vi "RTS Run Door Ops.vi"(5 "Delay":bool, 6 "Relay Number":u8=1 min=1 max=3 step=1, 7 "Station 1-8 Data in":T1 {"Station Slide"."Chamber 1-1"."Start Time" format="%<%X\n%x>T"; "Station Slide"."Chamber 1-1"."End Time" format="%<%X\n%x>T"; "Station Slide"."Time Count (s)" format="%.2f"; "Station Cab"."Chamber 1-1"."Start Time" format="%<%X\n%x>T"; "Station Cab"."Chamber 1-1"."End Time" format="%<%X\n%x>T"; "Station Cab"."Time Count (s)" format="%.2f"; "Station Freezer"."Chamber 1-1"."Start Time" format="%<%X\n%x>T"; "Station Freezer"."Chamber 1-1"."End Time" format="%<%X\n%x>T"; "Station Freezer"."Time Count (s)" format="%.2f"}, 8 "Error In":errorcluster, 9 "Door Open Sequence:":T5, 10 "Complete?":bool, 11 "Current Status":string[](array[string])) -> (0 "Error Out":errorcluster, 1 "Door Open Sequence: Out":T5, 3 "Run Door Ops":bool)   [LabVIEW 2016]
uses:
  Type Definitions/RTS Door Ops Sequence.ctl
  Type Definitions/RTS Station Relay Ops.ctl
  Type Definitions/RTS Door Opener Indicator.ctl
  Type Definitions/RTS Door Ops Client.ctl
  Type Definitions/RTS Door Opening Schedule.ctl
panel:
  # "Chamber Conditions:"
  # "Chamber Conditions:"
  # "Chamber Conditions:"
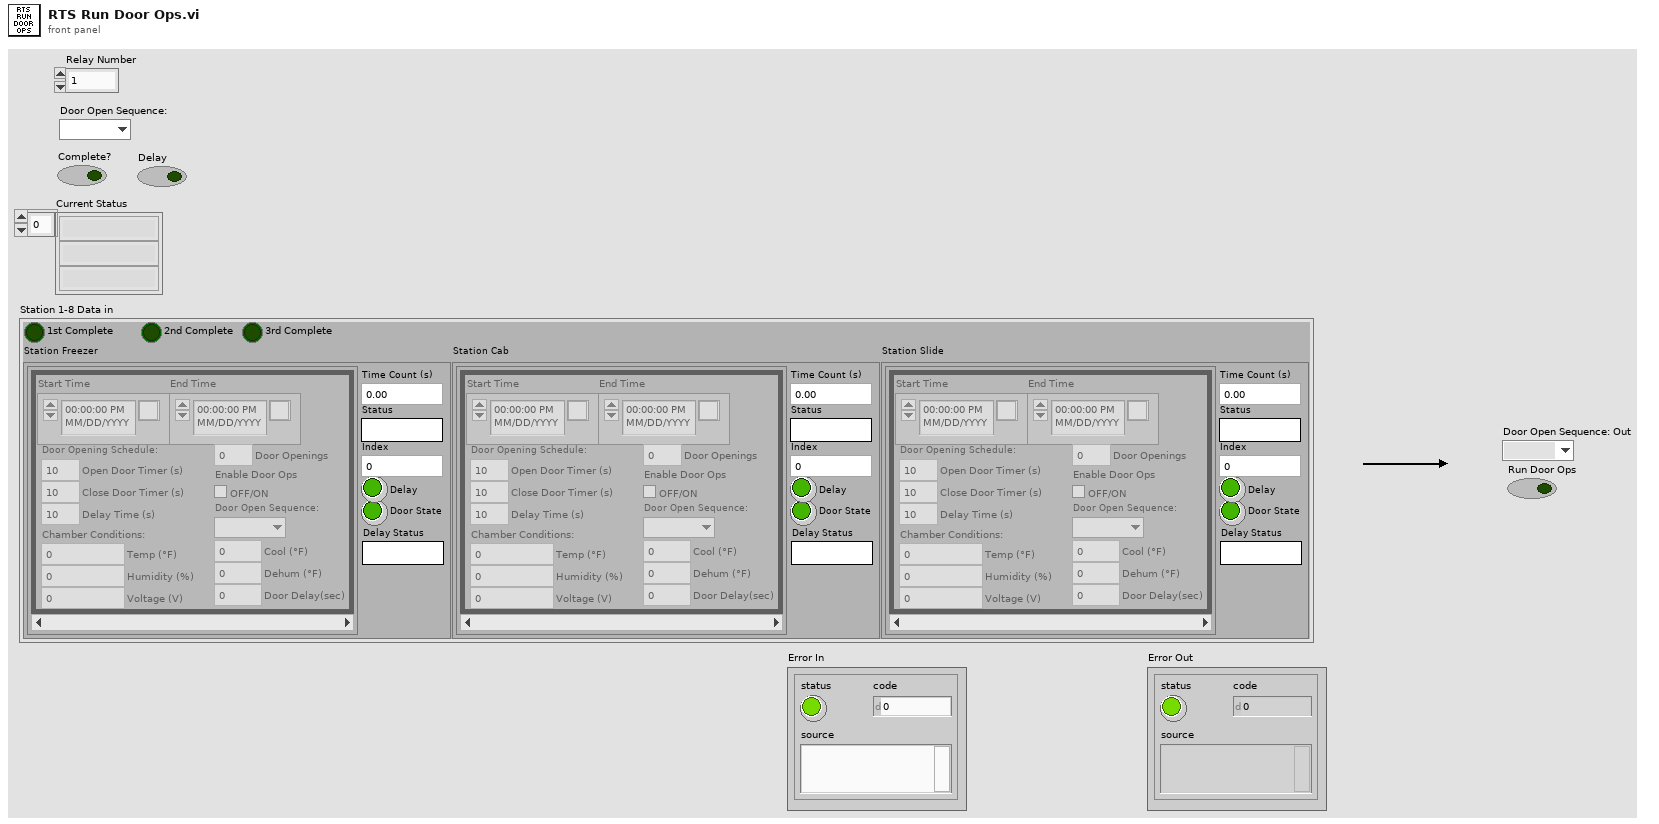
[diagram p1: front panel]
types:
  T1 = typedef "RTS Station Relay Ops.ctl" = cluster{"Station Freezer":T2, "Station Cab":T2, "Station Slide":T2, "1st Complete":bool, "2nd Complete":bool, "3rd Complete":bool}
  T2 = typedef "RTS Door Opener Indicator.ctl" = cluster{"Time Count (s)":dbl, "Status":string, "Door State":bool, "Delay":bool, "Chamber 1-1":T3[], "Index":i32, "Delay Status":string}
  T3 = typedef "RTS Door Ops Client.ctl" = cluster{"End Time":timestamp, "Start Time":timestamp, "Door Opening Schedule:":T4, "Enable Door Ops":bool, "Door Openings":u32, "Temp (°F)":dbl, "Humidity (%)":dbl, "Voltage (V)":dbl, "Door Open Sequence:":T5, "Door Delay(sec)":dbl, "Dehum (°F)":dbl, "Cool (°F)":dbl}
  T4 = typedef "RTS Door Opening Schedule.ctl" = cluster{"Open Door Timer (s)":dbl, "Delay Time (s)":dbl, "Close Door Timer (s)":dbl}
  T5 = typedef "RTS Door Ops Sequence.ctl" = enum16{"", "1st", "2nd", "3rd"}
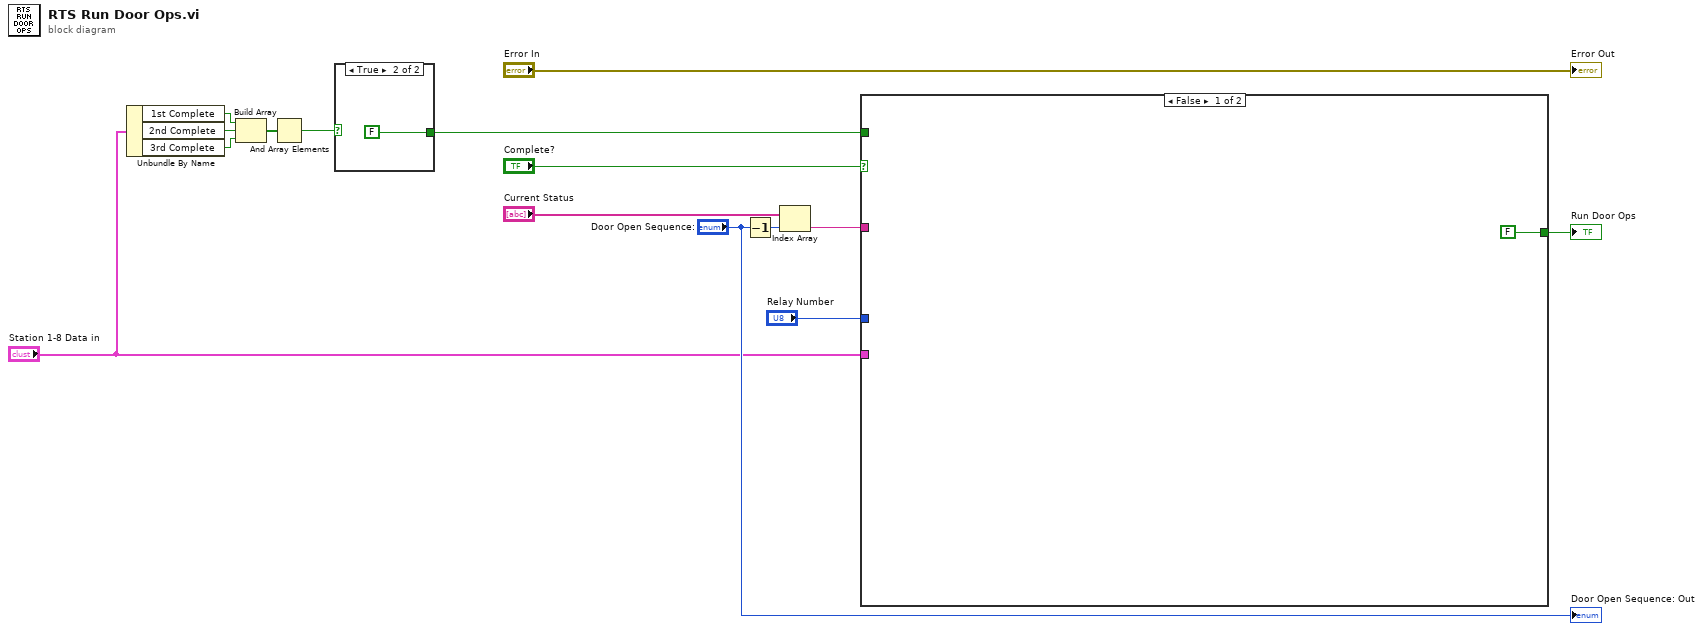
[diagram p0: block diagram]
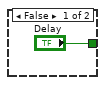
[diagram p2: hidden frame]
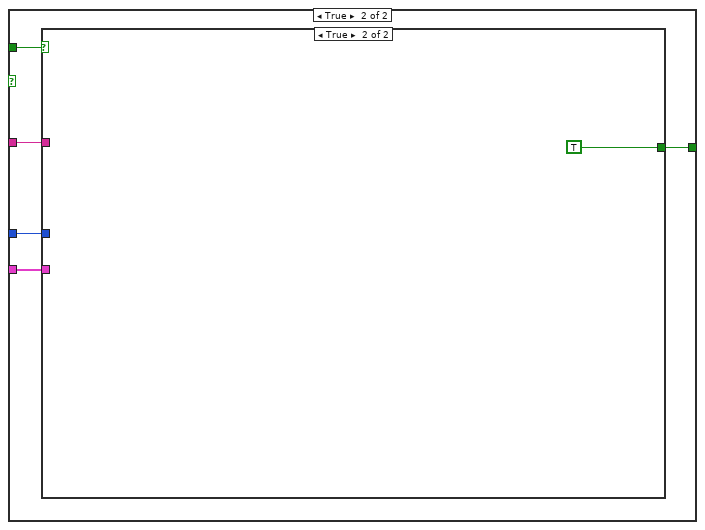
[diagram p3: hidden frame]
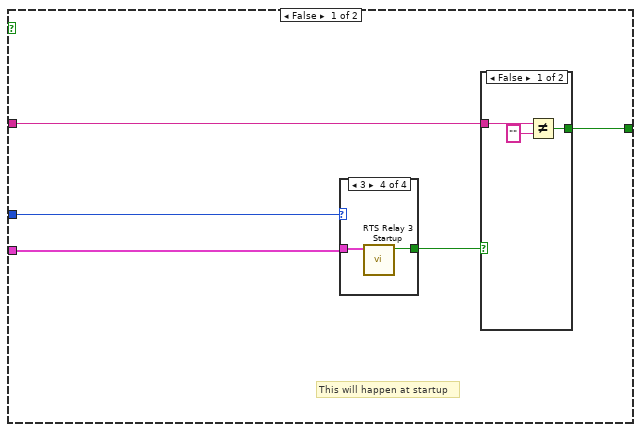
[diagram p4: hidden frame]
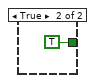
[diagram p5: hidden frame]
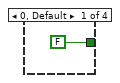
[diagram p6: hidden frame]
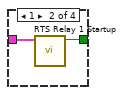
[diagram p7: hidden frame]
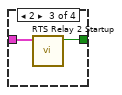
[diagram p8: hidden frame]
diagram:
  n1 = Unbundle By Name("Station 1-8 Data in") -> ("1st Complete"=w7:bool, "2nd Complete"=w6:bool, "3rd Complete"=w5:bool)
  n2 = Build Array(w7, w6, w5) -> (w4:bool[])
  n3 = And Array Elements(Boolean array=w4) -> (logical AND=w3:bool)
  n4 = case shown="True" w3 {
    tunnel: ["Delay" FALSE ("Delay")] -> w9
    frame False {
    }
    frame True {
    }
  }
  n5 = Decrement(x="Door Open Sequence:") -> (x-1=w11:T5)
  n6 = Index Array(array="Current Status", index=w11) -> (element=w15:string)
  n7 = case shown="False" "Complete?" {
    tunnel: [FALSE w22] -> w14
    tunnel: w15 -> [_ w23]
    tunnel: w9 -> [_ w21]
    tunnel: "Station 1-8 Data in" -> [_ w20]
    tunnel: "Relay Number" -> [_ w19]
    frame False {
    }
    frame True {
      n8 = case shown="True" w21 {
        tunnel: w23 -> [w28 _]
        tunnel: [w27 TRUE] -> w22
        tunnel: w20 -> [w25 _]
        tunnel: w19 -> [w24 _]
        frame False {
          # "This will happen at startup"
          n9 = case shown="3" w24 {
            tunnel: w25 -> [_ w34 w36 w38]
            tunnel: [FALSE w35 w37 w39] -> w26
            frame 0, Default {
            }
            frame 1 {
              n10 = call "RTS Relay 1 Startup.vi"("Station 1-8 Data in"=w34) -> ("Run Door Ops"=w35:bool)  [unwired: 10 in]
            }
            frame 2 {
              n11 = call "RTS Relay 2 Startup.vi"("Station 1-8 Data in"=w36) -> ("Run Door Ops"=w37:bool)  [unwired: 10 in]
            }
            frame 3 {
              n12 = call "RTS Relay 3 Startup.vi"("Station 1-8 Data in"=w38) -> ("Run Door Ops"=w39:bool)  [unwired: 10 in]
            }
          }
          n13 = case shown="False" w26 {
            tunnel: w28 -> [w30 _]
            tunnel: [w29 TRUE] -> w27
            frame False {
              n14 = Not Equal?(x=w30, y="") -> (x != y?=w29:bool)
            }
            frame True {
            }
          }
        }
        frame True {
        }
      }
    }
  }
  "Run Door Ops" <- w14
  "Error Out" <- "Error In"
  "Door Open Sequence: Out" <- "Door Open Sequence:"
